vi "PIM Handle Test Complete.vi"(8 "error in (no error)":errorcluster, 9 "Done?":bool, 10 "Quickmode?":bool, 11 "CMD Q":refnum<queue>) -> (0 "error out":errorcluster)   [LabVIEW 2011]
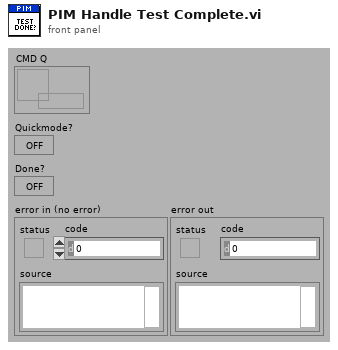
[diagram p1: front panel]
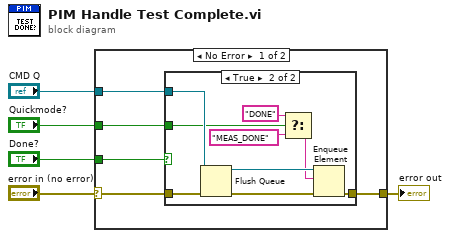
[diagram p0: block diagram]
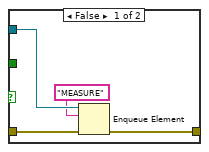
[diagram p2: hidden frame]
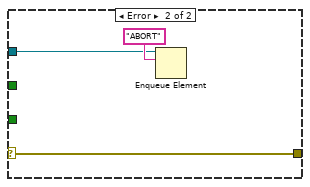
[diagram p3: hidden frame]
diagram:
  n1 = case shown="No Error" "error in (no error)" {
    selector: "error in (no error)" -> [w7 w26]
    tunnel: "Quickmode?" -> [w6 _]
    tunnel: "CMD Q" -> [w10 w24]
    tunnel: [w9 w26] -> w3
    tunnel: "Done?" -> [w8 _]
    frame No Error {
      n2 = case shown="True" w8 {
        tunnel: w10 -> [w12 w22]
        tunnel: w7 -> [w14 w21]
        tunnel: [w13 w19] -> w9
        tunnel: w6 -> [_ w16]
        frame False {
          n3 = Enqueue Element(queue=w12, element="MEASURE", error in (no error)=w14) -> (error out=w13:errorcluster)  [unwired: 3 out]
        }
        frame True {
          n4 = Flush Queue(queue=w22, error in (no error)=w21) -> (queue out=w23:refnum<queue>, error out=w20:errorcluster)  [unwired: 1 out]
          n5 = Select(t="DONE", s=w16, f="MEAS_DONE") -> (s? t:f=w15:string)
          n6 = Enqueue Element(queue=w23, element=w15, error in (no error)=w20) -> (error out=w19:errorcluster)  [unwired: 3 out]
        }
      }
    }
    frame Error {
      n7 = Enqueue Element(queue=w24, element="ABORT") -> ()  [unwired: 1 in, 4 out]
    }
  }
  "error out" <- w3
